vi "test_libssh2_session_last_error.vi"() -> ()   [LabVIEW 2013, in "libssh2_integration_tests.lvlib"]
uses:
  libssh2_integration_tests.lvlib
  <vilib>/addons/_JKI Toolkits/Caraya/classes/Test/Test.lvclass
  <vilib>/addons/_JKI Toolkits/Caraya/classes/Assert/Assert.lvclass
  libssh2/libssh2.lvlib
panel:
  out "error out":errorcluster
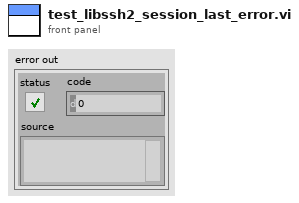
[diagram p1: front panel]
types:
  T1 = cluster{"error code":i32, "error message":string}[]
  T2 = typedef "libssh2.lvlib/Session Refnum.ctl" = refnum<k1>
  T3 = cluster{"error code":i32, "error message":string}
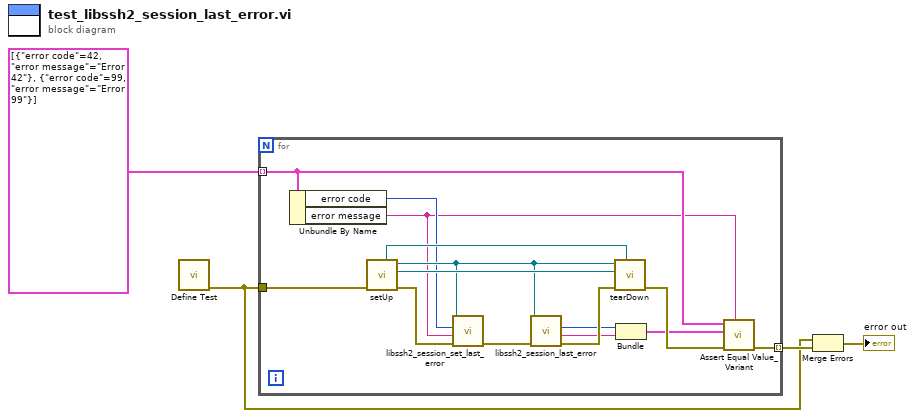
[diagram p0: block diagram]
diagram:
  n1 = call <vilib>:"Define Test.vi"() -> ("error out"=w2:errorcluster)  [unwired: 10 in, 1 out]
  n2 = for {
    tunnel: [w19] -> w4 mode=indexing
    tunnel: w2 -> [w18]
    tunnel: T1 [{"error code"=42, "error message"="Error 42"}, {"error code"=99, "error message"="Error 99"}] -> [w6] mode=indexing
    n3 = Unbundle By Name(w6) -> ("error code"=w10:i32, "error message"=w5:string)
    n4 = call "setUp.vi"("error in (no error)"=w18) -> ("error out"=w14:errorcluster, "connection ID"=w17:refnum<k5>, "session"=w11:T2, "fixture"=w16:refnum<class "Server Fixture.lvclass">)  [unwired: 7 in]
    n5 = call "libssh2_session_set_last_error.vi"("error in (no error)"=w14, "error message"=w5, "error code"=w10, "session"=w11) -> ("error out"=w15:errorcluster)  [unwired: 7 in]
    n6 = call "libssh2_session_last_error.vi"("error in (no error)"=w15, "session"=w11) -> ("error out"=w12:errorcluster, "error message"=w8:string, "error code"=w9:i32)  [unwired: 7 in]
    n7 = call "tearDown.vi"("fixture"=w16, "error in (no error)"=w12, "connection ID"=w17, "session"=w11) -> ("error out"=w13:errorcluster)  [unwired: 7 in]
    n8 = Bundle("error code"=w9, "error message"=w8) -> (w7:T3)  [unwired: 1 in]
    n9 = call <vilib>:"Assert Equal Value_Variant.vi"("Label"=w5, "error in (no error)"=w13, "Y"=w7, "X"=w6) -> ("error out"=w19:errorcluster)  [unwired: 6 in, 1 out]
  }
  n10 = Merge Errors(w2, w4) -> (→"error out":errorcluster)
